vi "Arm to Pickup Position.vi"(7 "Description":string, 8 "Command Info In":T1) -> (0 "Command Info Out":T1)   [LabVIEW 2019]
doc: "This template is useful for immediate subsystem actions that do not need deadband filtering\n\nBe sure to right-click and select New from Template and save with a new command name."
uses:
  <vilib>/Rock Robotics/WPI/Framework/Command Status Info.ctl
  <vilib>/Rock Robotics/WPI/Framework/Completion Status.ctl
  <vilib>/Rock Robotics/WPI/Framework/Completion Notifier.ctl
  Implementation/Arm Setpoints.ctl
  Implementation/Arm Operations.ctl
panel:
  in  "Down Position":dbl=-10.0
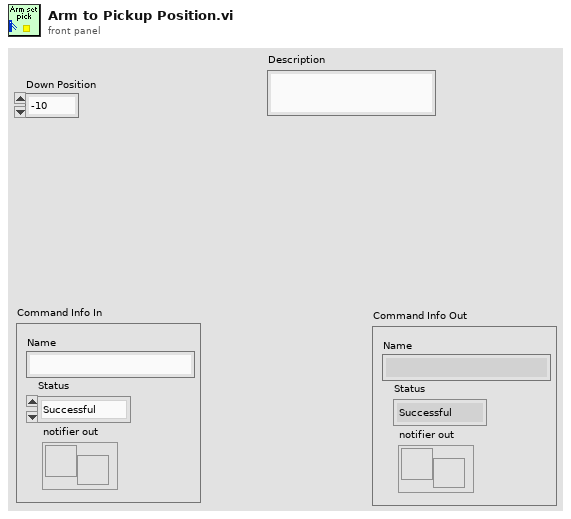
[diagram p1: front panel]
types:
  T1 = typedef "Command Status Info.ctl" = cluster{"Name":string, "Status":T2, "notifier out":T3}
  T2 = typedef "Completion Status.ctl" = enum16{"Successful", "Aborted", "Incomplete"}
  T3 = typedef "Completion Notifier.ctl" = refnum<notifier>
  T4 = typedef "Arm Setpoints.ctl" = cluster{"Operation":T5, "Setpoint":dbl, "Duration":dbl}
  T5 = typedef "Arm Operations.ctl" = enum16{"Reserve", "Read Current", "Turn to angle ", "Set position", "Immediate"}
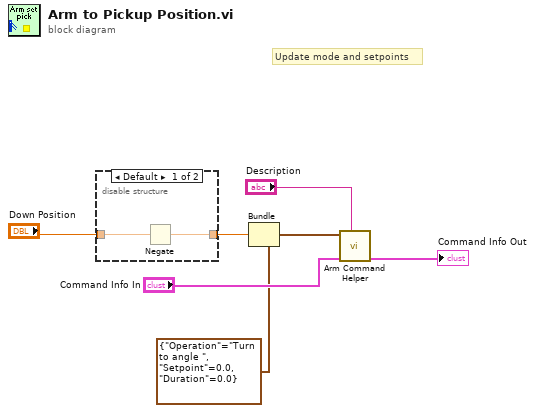
[diagram p0: block diagram]
diagram:
  # "Update mode and setpoints"
  n1 = disable-structure shown="Default" {
    disable-tunnel: "Down Position" -> [w9 w10]
    disable-tunnel: [w8 w10] -> w1
    frame condition #0 {
      n2 = Negate(x=w9) -> (-x=w8:dbl)
    }
    frame condition #1 (active) {
    }
  }
  n3 = Bundle(cluster=T4 {"Operation"=enum."Turn to angle ", "Setpoint"=0.0, "Duration"=0.0} ("SubSystem Data"), "Setpoint"=w1) -> (w2:T4)  [unwired: 2 in]
  n4 = call "Arm Command Helper.vi"("Description"="Description", "Command Info In"="Command Info In", "SubSystem Data"=w2) -> ("Command Info Out"=→"Command Info Out":T1)  [unwired: 6 in, 2 out]
